vi "YAFTAF_SetPersistentConfiguration.vi"(8 "ErrorIn":errorcluster, 10 "CmdData":variant, 11 "LocalIn":refnum<class>) -> (0 "ErrorOut":errorcluster, 2 "ReplyData":variant, 3 "LocalIn":refnum<class>, 4 "Exit":bool)   [LabVIEW 2021, in "YAFTAF.lvclass"]
uses:
  YAFTAF.lvclass
  YAFTAF.lvclass/YAFTAF.ctl
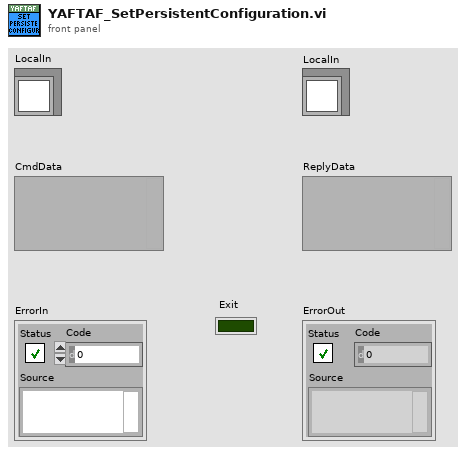
[diagram p1: front panel]
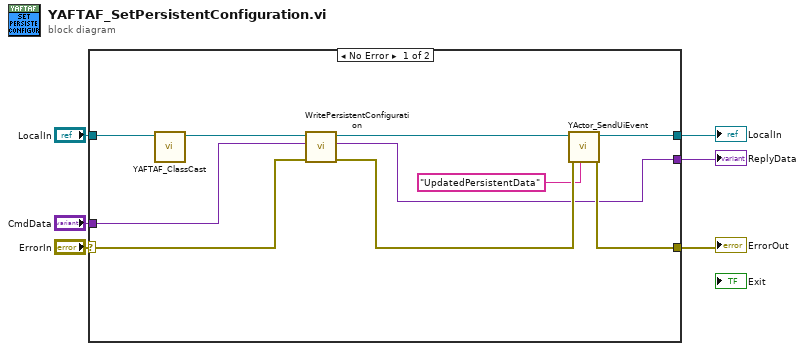
[diagram p0: block diagram]
diagram:
  n1 = case shown="No Error" "ErrorIn" {
    selector: "ErrorIn" -> [w16 w19]
    tunnel: [w14 w19] -> w5
    tunnel: [w8 w18] -> w3
    tunnel: "CmdData" -> [w9 w18]
    tunnel: "LocalIn" -> [w13 w17]
    tunnel: [w12 w17] -> w1
    frame No Error {
      n2 = call "YAFTAF_ClassCast.vi"("LocalIn"=w13) -> ("LocalOut"=w11:refnum<class "YAFTAF.lvclass">)  [unwired: 10 in]
      n3 = call-dynamic "WritePersistentConfiguration.vi"("ErrorIn"=w16, "DataIn"=w9, "ObjectIn"=w11) -> ("ErrorOut"=w15:errorcluster, "DataOut"=w8:variant, "ObjectOut"=w10:refnum<class "YAFTAF.lvclass">)  [unwired: 6 in]
      n4 = call-dynamic "YActor_SendUiEvent.vi"("Event"="UpdatedPersistentData", "ErrorIn"=w15, "YActorIn"=w10) -> ("ErrorOut"=w14:errorcluster, "YActorOut"=w12:refnum<class "YAFTAF.lvclass">)  [unwired: 7 in]
    }
    frame Error {
    }
  }
  "ErrorOut" <- w5
  "LocalIn" <- w1
  "ReplyData" <- w3
